vi "niFpgaHtCmulSimTemplate.vi"(0 "xr":fxp<+/-,31,31>, 5 "xi":fxp<+/-,31,31>, 7 "yr":fxp<+/-,31,31>, 9 "yi":fxp<+/-,31,31>, 11 "input valid":bool=TRUE, 12 "ready for output":bool=TRUE) -> (4 "pr":fxp<+/-,63,63>, 6 "pi":fxp<+/-,63,63>, 10 "overflow":bool, 14 "ready for input":bool, 15 "output valid":bool)   [LabVIEW 2017]
uses:
  <vilib>/rvi/FXPMathLib/SharedSubVIs/typedef/nifxpmath_BASIC_ImplementationSettings.ctl
  <vilib>/fxp/LVFixedPointQuantizationPolicyTypeDef.ctl
  <vilib>/fxp/LVFixedPointOverflowPolicyTypeDef.ctl
  <vilib>/rvi/ClientSDK/Core/DevComputerLib/niFpgaDevCompUtilities.lvlib
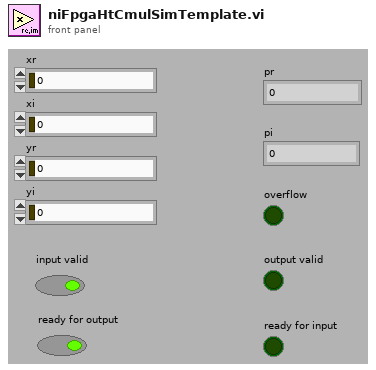
[diagram p1: front panel]
types:
  T1 = typedef "nifxpmath_BASIC_ImplementationSettings.ctl" = cluster{"NumOfStages":i32, "SupportSCTL":bool, "InputRegister":bool, "OutputRegister":bool, "rounding mode":T2, "overflow mode":T3}
  T2 = typedef "LVFixedPointQuantizationPolicyTypeDef.ctl" = enum32{"Truncate", "Round-Half-Up (Asymmetric)", "Round-Half-Even"}
  T3 = typedef "LVFixedPointOverflowPolicyTypeDef.ctl" = enum32{"Wrap", "Saturate"}
  T4 = typedef "niFpgaDevCompUtilities.lvlib/Cint64.ctl" = cluster{"real":i64, "imag":i64, "pr ovfl":bool, "pi ovfl":bool, "op ovfl":bool}
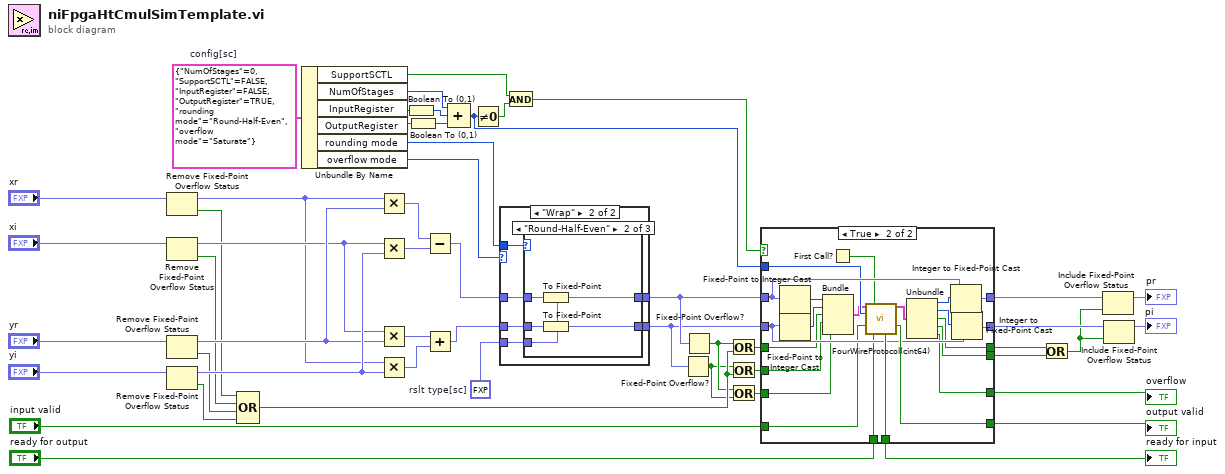
[diagram p0: block diagram]
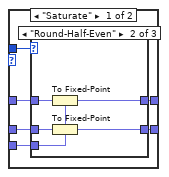
[diagram p3: hidden frame]
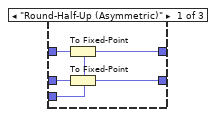
[diagram p4: hidden frame]
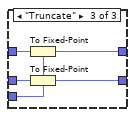
[diagram p5: hidden frame]
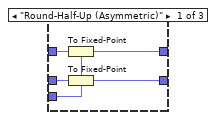
[diagram p6: hidden frame]
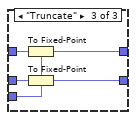
[diagram p7: hidden frame]
diagram:
  w21 = fxp<+/-,63,63> 0.0  # rslt type[sc]
  w46 = T1 {"NumOfStages"=0, "SupportSCTL"=FALSE, "InputRegister"=FALSE, "OutputRegister"=TRUE, "rounding mode"=enum."Round-Half-Even", "overflow mode"=enum."Saturate"}  # config[sc]
  n1 = Remove Fixed-Point Overflow Status(3:"xr") -> (0:w36:bool, 1:w37:fxp<+/-,31,31>)
  n2 = Remove Fixed-Point Overflow Status(3:"xi") -> (0:w35:bool, 1:w38:fxp<+/-,31,31>)
  n3 = Remove Fixed-Point Overflow Status(3:"yr") -> (0:w34:bool, 1:w39:fxp<+/-,31,31>)
  n4 = Remove Fixed-Point Overflow Status(3:"yi") -> (0:w33:bool, 1:w40:fxp<+/-,31,31>)
  n5 = Compound Arithmetic op=OR(w36, w35, w34, w33) -> (w18:bool)
  n6 = Unbundle By Name(w46) -> ("SupportSCTL"=w45:bool, "NumOfStages"=w24:i32, "InputRegister"=w26:bool, "OutputRegister"=w25:bool, "rounding mode"=w20:T2, "overflow mode"=w19:T3)
  n7 = Multiply(x=w37, y=w39) -> (x*y=w10:fxp<+/-,62,62>)
  n8 = Multiply(x=w38, y=w40) -> (x*y=w11:fxp<+/-,62,62>)
  n9 = Multiply(x=w38, y=w39) -> (x*y=w13:fxp<+/-,62,62>)
  n10 = Multiply(x=w37, y=w40) -> (x*y=w12:fxp<+/-,62,62>)
  n11 = Boolean To (0,1)(Boolean=w26) -> (0, 1=w28:i16)
  n12 = Boolean To (0,1)(Boolean=w25) -> (0, 1=w27:i16)
  n13 = Subtract(x=w10, y=w11) -> (x-y=w8:fxp<+/-,62,62>)
  n14 = Add(x=w13, y=w12) -> (x+y=w9:fxp<+/-,63,63>)
  n15 = Compound Arithmetic op=unknown(w24, w28, w27) -> (w22:i32)
  n16 = Not Equal To 0?(x=w22) -> (x != 0?=w23:bool)
  n17 = case shown="\"Wrap\"" w19 {
    tunnel: w8 -> [w57 w73]
    tunnel: w9 -> [w52 w78]
    tunnel: [w56 w77] -> w7
    tunnel: [w55 w76] -> w6
    tunnel: w21 -> [w54 w75]
    tunnel: w20 -> [w53 w74]
    frame "Saturate" {
      n18 = case shown="\"Round-Half-Even\"" w53 {
        tunnel: w57 -> [w62 w67 w72]
        tunnel: w52 -> [w61 w66 w71]
        tunnel: [w60 w65 w70] -> w56
        tunnel: [w59 w64 w69] -> w55
        tunnel: w54 -> [w58 w63 w68]
        frame "Round-Half-Up (Asymmetric)" {
          n19 = To Fixed-Point(fixed-point type=w58, number=w62) -> (fixed-point=w60:fxp<+/-,63,63>)
          n20 = To Fixed-Point(fixed-point type=w58, number=w61) -> (fixed-point=w59:fxp<+/-,63,63>)
        }
        frame "Round-Half-Even" {
          n21 = To Fixed-Point(fixed-point type=w63, number=w67) -> (fixed-point=w65:fxp<+/-,63,63>)
          n22 = To Fixed-Point(fixed-point type=w63, number=w66) -> (fixed-point=w64:fxp<+/-,63,63>)
        }
        frame "Truncate" {
          n23 = To Fixed-Point(fixed-point type=w68, number=w72) -> (fixed-point=w70:fxp<+/-,63,63>)
          n24 = To Fixed-Point(fixed-point type=w68, number=w71) -> (fixed-point=w69:fxp<+/-,63,63>)
        }
      }
    }
    frame "Wrap" {
      n25 = case shown="\"Round-Half-Even\"" w74 {
        tunnel: w78 -> [w82 w87 w93]
        tunnel: [w81 w86 w92] -> w77
        tunnel: [w80 w85 w91] -> w76
        tunnel: w75 -> [w79 w84 w90]
        tunnel: w73 -> [w83 w88 w89]
        frame "Round-Half-Up (Asymmetric)" {
          n26 = To Fixed-Point(fixed-point type=w79, number=w83) -> (fixed-point=w81:fxp<+/-,63,63>)
          n27 = To Fixed-Point(fixed-point type=w79, number=w82) -> (fixed-point=w80:fxp<+/-,63,63>)
        }
        frame "Round-Half-Even" {
          n28 = To Fixed-Point(fixed-point type=w84, number=w88) -> (fixed-point=w86:fxp<+/-,63,63>)
          n29 = To Fixed-Point(fixed-point type=w84, number=w87) -> (fixed-point=w85:fxp<+/-,63,63>)
        }
        frame "Truncate" {
          n30 = To Fixed-Point(fixed-point type=w90, number=w89) -> (fixed-point=w92:fxp<+/-,63,63>)
          n31 = To Fixed-Point(fixed-point type=w90, number=w93) -> (fixed-point=w91:fxp<+/-,63,63>)
        }
      }
    }
  }
  n32 = And(x=w45, y=w23) -> (x .and. y?=w44:bool)
  n33 = Fixed-Point Overflow?(1:w6) -> (0:w4:bool)
  n34 = Fixed-Point Overflow?(1:w7) -> (0:w5:bool)
  n35 = Or(x=w5, y=w18) -> (x .or. y?=w3:bool)
  n36 = Or(x=w4, y=w18) -> (x .or. y?=w2:bool)
  n37 = Or(x=w5, y=w4) -> (x .or. y?=w1:bool)
  n38 = case shown="True" w44 {
    tunnel: [_ w120] -> w48
    tunnel: [_ w119] -> w47
    tunnel: w7 -> [w98 w112]
    tunnel: w6 -> [w97 w111]
    tunnel: [w98 w115] -> w32
    tunnel: [w97 w113] -> w30
    tunnel: "input valid" -> [_ w110]
    tunnel: "ready for output" -> [_ w109]
    tunnel: w22 -> [_ w107]
    tunnel: [w96 w105] -> w16
    tunnel: w3 -> [w96 w103]
    tunnel: w2 -> [w95 w102]
    tunnel: w1 -> [w94 w101]
    tunnel: [w95 w100] -> w15
    tunnel: [w94 w99] -> w17
    frame False {
    }
    frame True {
      n39 = Fixed-Point to Integer Cast(1:w112) -> (0:w117:i64)
      n40 = Fixed-Point to Integer Cast(1:w111) -> (0:w118:i64)
      n41 = Bundle(w117, w118, w103, w102, w101) -> (w104:cluster{i64, i64, bool, bool, bool})  [unwired: 1 in]
      n42 = First Call?() -> (First Call?: T/F=w108:bool)
      n43 = call <vilib>:"FourWireProtocol(cint64).vi"("complex data in"=w104, "reset"=w108, "latency (1)"=w107, "input valid"=w110, "ready for output"=w109) -> ("complex data out"=w106:T4, "output valid"=w119:bool, "ready for input"=w120:bool)  [unwired: 7 in, 1 out]
      n44 = Unbundle(w106) -> ("real"=w116:i64, "imag"=w114:i64, "pr ovfl"=w105:bool, "pi ovfl"=w100:bool, "op ovfl"=w99:bool)
      n45 = Integer to Fixed-Point Cast(fixed-point type=w112, integer=w116) -> (fixed-point=w115:fxp<+/-,63,63>)
      n46 = Integer to Fixed-Point Cast(fixed-point type=w111, integer=w114) -> (fixed-point=w113:fxp<+/-,63,63>)
    }
  }
  "output valid" <- w47
  "ready for input" <- w48
  "overflow" <- w17
  n47 = Or(x=w16, y=w15) -> (x .or. y?=w14:bool)
  n48 = Include Fixed-Point Overflow Status(2:w14, 3:w32) -> (1:→"pr":fxp<+/-,63,63>)
  n49 = Include Fixed-Point Overflow Status(2:w14, 3:w30) -> (1:→"pi":fxp<+/-,63,63>)
